vi "Close Splitter.vi"(8 "error in (no error)":errorcluster, 11 "Interaction Splitter in":refnum<class "Interaction Splitter.lvclass">) -> (0 "error out":errorcluster)   [LabVIEW 2021, in "Interaction Splitter.lvclass"]
doc: "Copyright 2018, Wiebe Walstra, wiebe@carya.nl."
uses:
  Interaction Splitter.lvclass
  Interaction Splitter.lvclass/Interaction Splitter.ctl
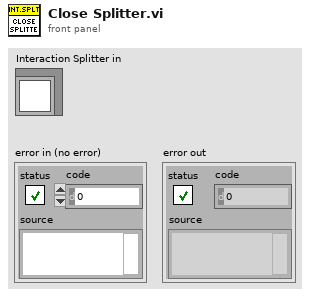
[diagram p1: front panel]
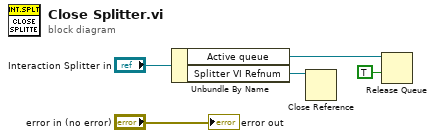
[diagram p0: block diagram]
diagram:
  n1 = Unbundle By Name("Interaction Splitter in") -> ("Active queue"=w2:refnum<queue>, "Splitter VI Refnum"=w3:refnum<vi>)
  n2 = Close Reference(reference=w3) -> ()  [unwired: 1 in, 1 out]
  n3 = Release Queue(queue=w2, force destroy? (F)=TRUE) -> ()  [unwired: 1 in, 3 out]
  "error out" <- "error in (no error)"
